vi "VI Server_Set Menu Ring by Item Selected.vi"(7 "Label":string, 8 "error in":errorcluster, 9 "Item":string, 11 "VI Server Cluster":T1) -> (0 "error out":errorcluster, 1 "Control Reference":refnum<vi>, 3 "VI Server Cluster.DUP":T1)   [LabVIEW 2020, in "VI Server Toolkit LV2013.lvlib"]
doc: "Sets value of Menu Ring by its item name/selection."
uses:
  VI Server Toolkit LV2013.lvlib
  VI Server_TypeDefs/VI Server_RefsCluster.ctl
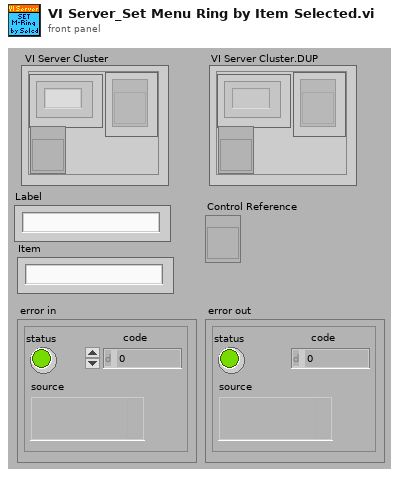
[diagram p1: front panel]
types:
  T1 = typedef "VI Server_RefsCluster.ctl" = cluster{"Labels":string[], "Refs":refnum<vi>[], "VI Ref":refnum<vi>}
  T2 = typedef "LVStringsAndValuesArrayTypeDef_U16.ctl" = cluster{"String":string, "Value":u16}[]
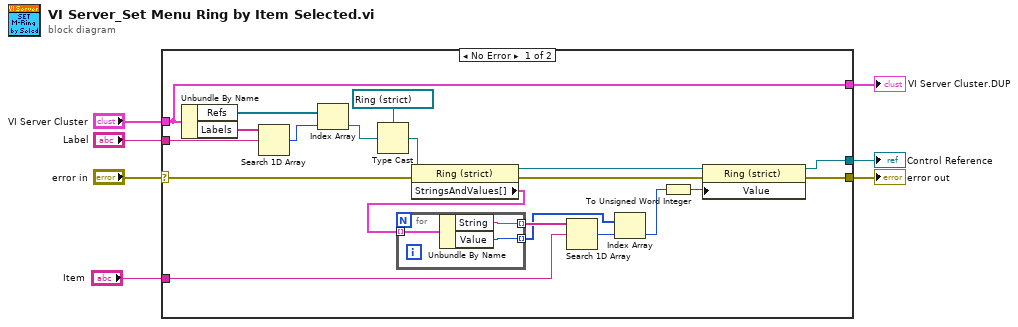
[diagram p0: block diagram]
diagram:
  n1 = case shown="No Error" "error in" {
    selector: "error in" -> [w22 w31]
    tunnel: "Label" -> [w26 _]
    tunnel: "VI Server Cluster" -> [w9 _]
    tunnel: [w19 w31] -> w7
    tunnel: [w16 _] -> w3
    tunnel: "Item" -> [w21 _]
    tunnel: [w9 _] -> w1
    frame No Error {
      n2 = Unbundle By Name(w9) -> ("Refs"=w24:refnum<vi>[], "Labels"=w27:string[])
      n3 = Search 1D Array(1D array=w27, element=w26) -> (index of element=w25:i32)  [unwired: 1 out]
      n4 = Index Array(array=w24, index=w25) -> (element=w23:refnum<vi>)
      n5 = Type Cast(type=refnum<vi> refnum ("Ring"), x=w23) -> (*(type *) &x=w17:refnum<vi>)
      n6 = property class="Ring (strict)"(reference=w17, error in=w22) -> (reference out=w18:refnum<vi>, error out=w20:errorcluster, "StringsAndValues[]"=w14:T2)
      n7 = for {
        tunnel: w14 -> [w30] mode=indexing
        tunnel: [w29] -> w13 mode=indexing
        tunnel: [w28] -> w12 mode=indexing
        n8 = Unbundle By Name(w30) -> ("String"=w29:string, "Value"=w28:u16)
      }
      n9 = Search 1D Array(1D array=w13, element=w21) -> (index of element=w11:i32)  [unwired: 1 out]
      n10 = Index Array(array=w12, index=w11) -> (element=w10:u16)
      n11 = To Unsigned Word Integer(number=w10) -> (unsigned 16bit integer=w15:u16)
      n12 = property class="Ring (strict)"(reference=w18, error in=w20, "Value"=w15) -> (reference out=w16:refnum<vi>, error out=w19:errorcluster)
    }
    frame Error {
    }
  }
  "error out" <- w7
  "VI Server Cluster.DUP" <- w1
  "Control Reference" <- w3
